vi "256_to_10.vi"(1 "Array":i32[](array[numeric])) -> (0 "Numeric":dbl)   [LabVIEW 2015, in "Igor.lvclass"]
uses:
  Igor.lvclass
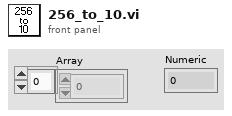
[diagram p1: front panel]
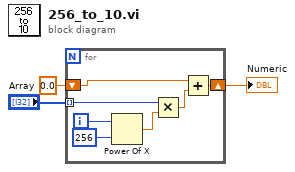
[diagram p0: block diagram]
diagram:
  n1 = for {
    tunnel: "Array" -> [w8] mode=indexing
    shift-right: [w5] -> w1
    shift-left: 0.0 -> [w4]
    i -> [w9]
    n2 = Power Of X(1:256 ("y"), 2:w9) -> (0:w7:dbl)
    n3 = Multiply(x=w8, y=w7) -> (x*y=w6:dbl)
    n4 = Add(x=w4, y=w6) -> (x+y=w5:dbl)
  }
  "Numeric" <- w1
